vi "Read_CmdRead.vi"(8 "error in (no error)":errorcluster, 11 "TcpServer in":refnum<class "TcpServer.lvclass">) -> (0 "error out":errorcluster, 2 "CmdRead":refnum<user-event>, 3 "TcpServer out":refnum<class "TcpServer.lvclass">)   [LabVIEW 2018]
uses:
  TcpServer.lvclass
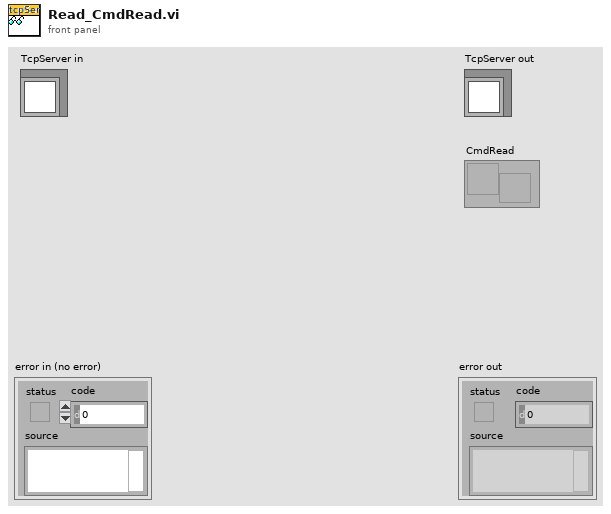
[diagram p1: front panel]
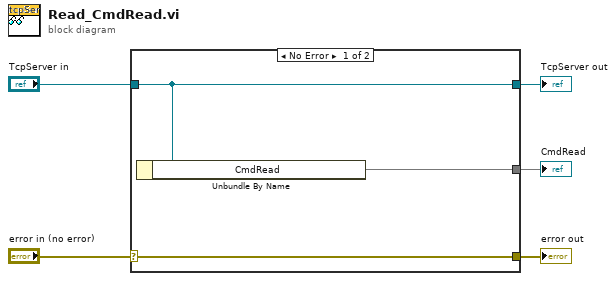
[diagram p0: block diagram]
diagram:
  n1 = case shown="No Error" "error in (no error)" {
    selector: "error in (no error)" -> [w8 w9]
    tunnel: [w8 w9] -> w4
    tunnel: [w7 w10] -> w2
    tunnel: "TcpServer in" -> [w7 w10]
    tunnel: [w6 _] -> w1
    frame No Error {
      n2 = Unbundle By Name(w7) -> ("CmdRead"=w6)
    }
    frame Error {
    }
  }
  "error out" <- w4
  "TcpServer out" <- w2
  "CmdRead" <- w1
